vi "Invoke Assertion.vi"() -> ()   [LabVIEW 2020, in "MacroAssert.lvlib"]
uses:
  MacroAssert.lvlib
panel:
  out "error out":errorcluster
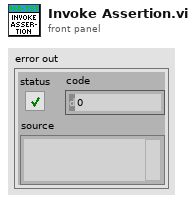
[diagram p1: front panel]
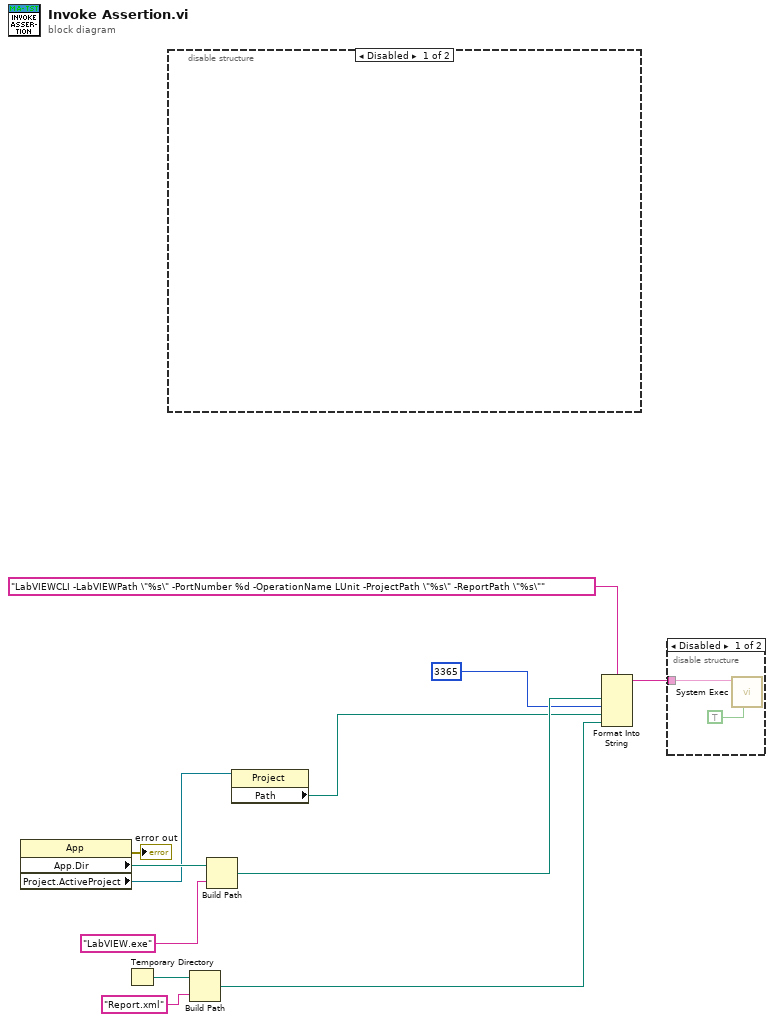
[diagram p0: block diagram]
diagram:
  n1 = property class="App"() -> (error out=→"error out":errorcluster, "App.Dir"=w12:path, "Project.ActiveProject"=w8:refnum<vi>)  [unwired: 2 in, 1 out]
  n2 = Temporary Directory() -> (w5:path)
  n3 = disable-structure shown="Disabled" {
    frame Disabled {
    }
    frame Enabled {
    }
  }
  n4 = Build Path(base path=w5, name or relative path="Report.xml") -> (appended path=w4:path)
  n5 = Build Path(base path=w12, name or relative path="LabVIEW.exe") -> (appended path=w9:path)
  n6 = property class="Project"(reference=w8) -> ("Path"=w7:path)  [unwired: 1 in, 2 out]
  n7 = Format Into String(format string="LabVIEWCLI -LabVIEWPath \"%s\" -PortNumber %d -OperationName LUnit -ProjectPath \"%s\" -ReportPath \"%s\"", w9, u32 3365 ("input 2"), w7, w4) -> (resulting string=w3:string)  [unwired: 2 in, 1 out]
  n8 = disable-structure shown="Disabled" {
    disable-tunnel: w3 -> [w13 _]
    frame Disabled {
      n9 = call <vilib>:"System Exec.vi"("run minimized? (F)"=TRUE, "command line"=w13) -> ()  [unwired: 6 in, 4 out]
    }
    frame Enabled {
    }
  }
